vi "HTML Dir.vi"(8 "error in (no error)":errorcluster) -> (0 "error out":errorcluster, 3 "path":path)   [LabVIEW 2014, in "lvprj2html.lvlib"]
uses:
  lvprj2html.lvlib
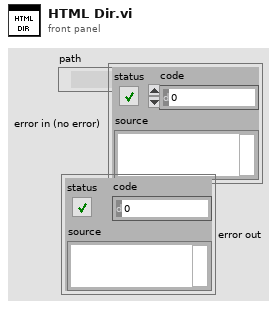
[diagram p1: front panel]
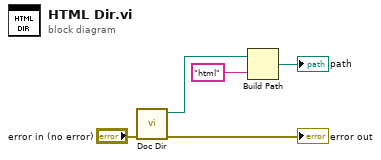
[diagram p0: block diagram]
diagram:
  n1 = call "Doc Dir.vi"("error in (no error)"="error in (no error)") -> ("error out"=→"error out":errorcluster, "appended path"=w3:path)  [unwired: 9 in]
  n2 = Build Path(base path=w3, name or relative path="html") -> (appended path=→"path":path)
